vi "Create Sections and Channels.vi"(8 "error in (no error)":errorcluster, 10 "Configuration":T1={"Name"="", "Description"="", "Diagnostics Basic Configuraiton"={"Database File"=path "", "CAN Interface"=enum."CAN0", "Baud Rate"=0, "Diagnostic Protocol"=enum."GMLAN", "Transport Protocol"=enum."ISO TP - Normal Mode", "Transmit ID"=0, "Receive ID"=0, "Transmit Extension"=0, "Receive Extension"=0, "Receive UUDT ID"=0, "Enable Stream"=TRUE, "VW TP Channel ID"=0, "Security"={"Source DLL Path"=path "", "Security Level"=1, "Target DLL Path"=path ""}, "Fill Frame"=FALSE, "Fill Byte"=255, "Termination"=FALSE}, "DIDs"={"Description"="", "Frames"=[]}, "Input PIDs"={"Description"="", "Frames"=[]}, "Output PIDs"={"Description"="", "Frames"=[]}, "DPIDs"={"Description"="", "DPIDs"=[]}, "DTC"={"Description"="", "DTC descriptor"={"DTC Byte Length"=2, "Status Byte Length"=1, "Add Data Byte Length"=1, "Byte Order"=enum."Motorola"}, "DTCControl"={"Description"="", "Signals"=[]}}, "NI 986x Support"={"Enable 986x"=FALSE, "RIO Device"=0, "Bitfile"=path ""}, "Commands"={"Description"=""}, "Status"={"Description"=""}, "IO Controls"={"Description"="", "IO Control Array"=[]}, "Routines"={"Description"="", "Routine Array"=[]}, "Output Memory"={"Description"="", "Frames"=[]}, "Input Memory"={"Description"="", "Frames"=[]}} {"Input Memory"."Frames"."Signals"."Byte Order" items=["Little Endian", "Big Endian"]; "Input Memory"."Frames"."Signals"."Data Type" items=["Signed", "Unsigned", "IEEE Float"]; "Output Memory"."Frames"."Signals"."Byte Order" items=["Little Endian", "Big Endian"]; "Output Memory"."Frames"."Signals"."Data Type" items=["Signed", "Unsigned", "IEEE Float"]; "Routines"."Routine Array"."Stop Parameters"."Response"."Byte Order" items=["Little Endian", "Big Endian"]; "Routines"."Routine Array"."Stop Parameters"."Response"."Data Type" items=["Signed", "Unsigned", "IEEE Float"]; "Routines"."Routine Array"."Stop Parameters"."Cmd"."Byte Order" items=["Little Endian", "Big Endian"]; "Routines"."Routine Array"."Stop Parameters"."Cmd"."Data Type" items=["Signed", "Unsigned", "IEEE Float"]; "Routines"."Routine Array"."Request Parameters"."Response"."Byte Order" items=["Little Endian", "Big Endian"]; "Routines"."Routine Array"."Request Parameters"."Response"."Data Type" items=["Signed", "Unsigned", "IEEE Float"]; "Routines"."Routine Array"."Request Parameters"."Cmd"."Byte Order" items=["Little Endian", "Big Endian"]; "Routines"."Routine Array"."Request Parameters"."Cmd"."Data Type" items=["Signed", "Unsigned", "IEEE Float"]; "Routines"."Routine Array"."Start Parameters"."Response"."Byte Order" items=["Little Endian", "Big Endian"]; "Routines"."Routine Array"."Start Parameters"."Response"."Data Type" items=["Signed", "Unsigned", "IEEE Float"]; "Routines"."Routine Array"."Start Parameters"."Cmd"."Byte Order" items=["Little Endian", "Big Endian"]; "Routines"."Routine Array"."Start Parameters"."Cmd"."Data Type" items=["Signed", "Unsigned", "IEEE Float"]; "IO Controls"."IO Control Array"."Signals"."Response"."Byte Order" items=["Little Endian", "Big Endian"]; "IO Controls"."IO Control Array"."Signals"."Response"."Data Type" items=["Signed", "Unsigned", "IEEE Float"]; "IO Controls"."IO Control Array"."Signals"."Cmd"."Byte Order" items=["Little Endian", "Big Endian"]; "IO Controls"."IO Control Array"."Signals"."Cmd"."Data Type" items=["Signed", "Unsigned", "IEEE Float"]; "DTC"."DTCControl"."Signals"."Byte Order" items=["Little Endian", "Big Endian"]; "DTC"."DTCControl"."Signals"."Data Type" items=["Signed", "Unsigned", "IEEE Float"]; "Diagnostics Basic Configuraiton"."Fill Byte" format="%.0x"; "Diagnostics Basic Configuraiton"."VW TP Channel ID" format="%.0x"; "Diagnostics Basic Configuraiton"."Receive UUDT ID" format="%.0x"; "Diagnostics Basic Configuraiton"."Receive Extension" format="%.0x"; "Diagnostics Basic Configuraiton"."Transmit Extension" format="%.0x"; "Diagnostics Basic Configuraiton"."Receive ID" format="%.0x"; "Diagnostics Basic Configuraiton"."Transmit ID" format="%.0x"; "DIDs"."Frames"."Signals"."Byte Order" items=["Little Endian", "Big Endian"]; "DIDs"."Frames"."Signals"."Data Type" items=["Signed", "Unsigned", "IEEE Float"]; "Input PIDs"."Frames"."Signals"."Byte Order" items=["Little Endian", "Big Endian"]; "Input PIDs"."Frames"."Signals"."Data Type" items=["Signed", "Unsigned", "IEEE Float"]; "Output PIDs"."Frames"."Signals"."Byte Order" items=["Little Endian", "Big Endian"]; "Output PIDs"."Frames"."Signals"."Data Type" items=["Signed", "Unsigned", "IEEE Float"]}, 11 "Device Item Ref in":T25 format="%.0x") -> (0 "error out":errorcluster, 3 "Device Item Ref out":T25 format="%.0x")   [LabVIEW 2015, in "Diagnostics Addon System Explorer.lvlib"]
uses:
  Diagnostics Addon System Explorer.lvlib
  Types/FG Action.ctl
  <vilib>/NI Veristand/Custom Device API/Custom Device Channel.ctl
  <vilib>/NI Veristand/Custom Device API/Custom Device API.lvlib
  <vilib>/NI Veristand/Custom Device API/Custom Device Channel Type.ctl
  Shared/SubVIs/GUID Lookup.vi
  Shared/Diagnostics Addon Shared.lvlib
  Types/Frame Type.ctl
  Shared/Types/Signal Parameters.ctl
  <vilib>/NI Veristand/Custom Device API/Custom Device Item Ref.ctl
  Shared/Types/Diagnostic Protocols.ctl
  Shared/Types/CAN Interface.ctl
  Shared/Types/DPID Periodic Rate.ctl
  Shared/Types/DPID Parameters.ctl
  Types/Exported DPIDs Cluster.ctl
  Types/Exported Frames Cluster.ctl
  Shared/Types/Transport Protocols.ctl
  Shared/Types/CAN Configuration.ctl
  <vilib>/Automotive Diagnostic Command Set/Diagnostic Protocols.llb/DTC Descriptor.ctl
  Types/Exported DTC Cluster.ctl
  Types/Exported 986x Support.ctl
  Types/Exported Command Cluster.ctl
  Types/Exported Status Cluster.ctl
  Types/Exported Configuration.ctl
  Shared/Types/Frame Parameters.ctl
  Types/Exported DPID Parameters.ctl
  Shared/Types/Security.ctl
  Shared/Types/IO Control Parameters.ctl
  Shared/Types/Exported IO Control Cluster.ctl
  Shared/Types/Command Response Signals.ctl
  Shared/Types/Routine Paramaters.ctl
  Shared/Types/Exported Routines Cluster.ctl
  Shared/Types/Exported DTC Control Cluster.ctl
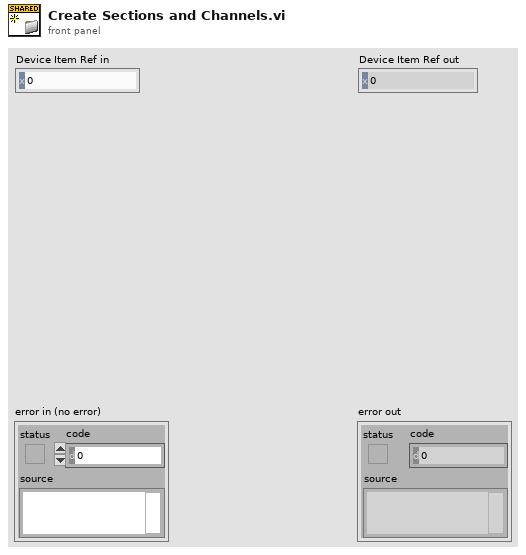
[diagram p1: front panel]
types:
  T1 = typedef "Diagnostics Addon System Explorer.lvlib/Exported Configuration.ctl" = cluster{"Name":string, "Description":string, "Diagnostics Basic Configuraiton":T2, "DIDs":T7, "Input PIDs":T7, "Output PIDs":T7, "DPIDs":T10, "DTC":T14, "NI 986x Support":T17, "Commands":T18, "Status":T19, "IO Controls":T20, "Routines":T23, "Output Memory":T7, "Input Memory":T7}
  T2 = typedef "Diagnostics Addon Shared.lvlib/CAN Configuration.ctl" = cluster{"Database File":path, "CAN Interface":T3, "Baud Rate":u32, "Diagnostic Protocol":T4, "Transport Protocol":T5, "Transmit ID":u32, "Receive ID":u32, "Transmit Extension":u8, "Receive Extension":u8, "Receive UUDT ID":u32, "Enable Stream":bool, "VW TP Channel ID":u32, "Security":T6, "Fill Frame":bool, "Fill Byte":u8, "Termination":bool}
  T3 = typedef "Diagnostics Addon Shared.lvlib/CAN Interface.ctl" = enum16{"CAN0", "CAN1", "CAN2", "CAN3", "CAN4", "CAN5", "CAN6", "CAN7", "CAN8", "CAN9", "CAN10", "CAN11", "CAN12", "CAN13", "CAN14", "CAN15", "CAN16", "CAN17", "CAN18", "CAN19", "CAN20", "CAN21", "CAN22", "CAN23", "CAN24", "CAN25", "CAN26", "CAN27", "CAN28", "CAN29", "CAN30", "CAN31", "CAN32", "CAN33", "CAN34", "CAN35", "CAN36", "CAN37", "CAN38", "CAN39", "CAN40", "CAN41", "CAN42", "CAN43", "CAN44", "CAN45", "CAN46", "CAN47", "CAN48", "CAN49", "CAN50", "CAN51", "CAN52", "CAN53", "CAN54", "CAN55", "CAN56", "CAN57", "CAN58", "CAN59", "CAN60", "CAN61", "CAN62", "CAN63", "CAN 256 (Virtual)", "CAN 257 (Virtual)"}
  T4 = typedef "Diagnostics Addon Shared.lvlib/Diagnostic Protocols.ctl" = enum16{"GMLAN", "KWP-2000", "UDS"}
  T5 = typedef "Diagnostics Addon Shared.lvlib/Transport Protocols.ctl" = enum16{"ISO TP - Normal Mode", "ISO TP - Mixed Mode", "VW TP 2.0", "Diagnostics on IP"}
  T6 = typedef "Diagnostics Addon Shared.lvlib/Security.ctl" = cluster{"Source DLL Path":path, "Security Level":u8, "Target DLL Path":path}
  T7 = typedef "Diagnostics Addon System Explorer.lvlib/Exported Frames Cluster.ctl" = cluster{"Description":string, "Frames":T8[]}
  T8 = typedef "Diagnostics Addon Shared.lvlib/Frame Parameters.ctl" = cluster{"Name":string, "Description":string, "ID":u32, "Signals":T9[]}
  T9 = typedef "Diagnostics Addon Shared.lvlib/Signal Parameters.ctl" = cluster{"Start Bit":u8, "Length":u8, "Scaling Factor":dbl, "Scaling Offset":dbl, "Minimum":dbl, "Maximum":dbl, "Data Type":u32, "Byte Order":u32, "Default Value":dbl, "Name":string, "Units":string, "Description":string}
  T10 = typedef "Diagnostics Addon System Explorer.lvlib/Exported DPIDs Cluster.ctl" = cluster{"Description":string, "DPIDs":T11[]}
  T11 = typedef "Diagnostics Addon System Explorer.lvlib/Exported DPID Parameters.ctl" = cluster{"Name":string, "Description":string, "DPID":T12}
  T12 = typedef "Diagnostics Addon Shared.lvlib/DPID Parameters.ctl" = cluster{"DPID ID":u8, "Speed":T13, "PIDs":u16[]}
  T13 = typedef "Diagnostics Addon Shared.lvlib/DPID Periodic Rate.ctl" = enum16{"Slow", "Medium", "Fast"}
  T14 = typedef "Diagnostics Addon System Explorer.lvlib/Exported DTC Cluster.ctl" = cluster{"Description":string, "DTC descriptor":T15, "DTCControl":T16}
  T15 = typedef "Diagnostics Addon Shared.lvlib/DTC Descriptor.ctl" = cluster{"DTC Byte Length":i32, "Status Byte Length":i32, "Add Data Byte Length":i32, "Byte Order":enum16{"Motorola", "Intel"}}
  T16 = typedef "Diagnostics Addon Shared.lvlib/Exported DTC Control Cluster.ctl" = cluster{"Description":string, "Signals":T9[]}
  T17 = typedef "Diagnostics Addon System Explorer.lvlib/Exported 986x Support.ctl" = cluster{"Enable 986x":bool, "RIO Device":u16, "Bitfile":path}
  T18 = typedef "Diagnostics Addon System Explorer.lvlib/Exported Command Cluster.ctl" = cluster{"Description":string}
  T19 = typedef "Diagnostics Addon System Explorer.lvlib/Exported Status Cluster.ctl" = cluster{"Description":string}
  T20 = typedef "Diagnostics Addon Shared.lvlib/Exported IO Control Cluster.ctl" = cluster{"Description":string, "IO Control Array":T21[]}
  T21 = typedef "Diagnostics Addon Shared.lvlib/IO Control Parameters.ctl" = cluster{"Name":string, "Description":string, "ID":u16, "Signals":T22}
  T22 = typedef "Diagnostics Addon Shared.lvlib/Command Response Signals.ctl" = cluster{"Cmd":T9[], "Response":T9[]}
  T23 = typedef "Diagnostics Addon Shared.lvlib/Exported Routines Cluster.ctl" = cluster{"Description":string, "Routine Array":T24[]}
  T24 = typedef "Diagnostics Addon Shared.lvlib/Routine Paramaters.ctl" = cluster{"Name":string, "Description":string, "ID":u16, "Start Parameters":T22, "Request Parameters":T22, "Stop Parameters":T22}
  T25 = typedef "Custom Device API.lvlib/Custom Device Item Ref.ctl" = u64
  T26 = typedef "Custom Device API.lvlib/Custom Device Channel.ctl" = cluster{"Type":T27, "Units":string, "Default Value":dbl, "Faultable":bool, "Scalable":bool}
  T27 = typedef "Custom Device API.lvlib/Custom Device Channel Type.ctl" = enum16{"Input", "Output"}
  T28 = typedef "Diagnostics Addon System Explorer.lvlib/FG Action.ctl" = enum16{"Get", "Set"}
  T29 = typedef "Diagnostics Addon System Explorer.lvlib/Frame Type.ctl" = enum8{"PID", "DID", "Memory"}
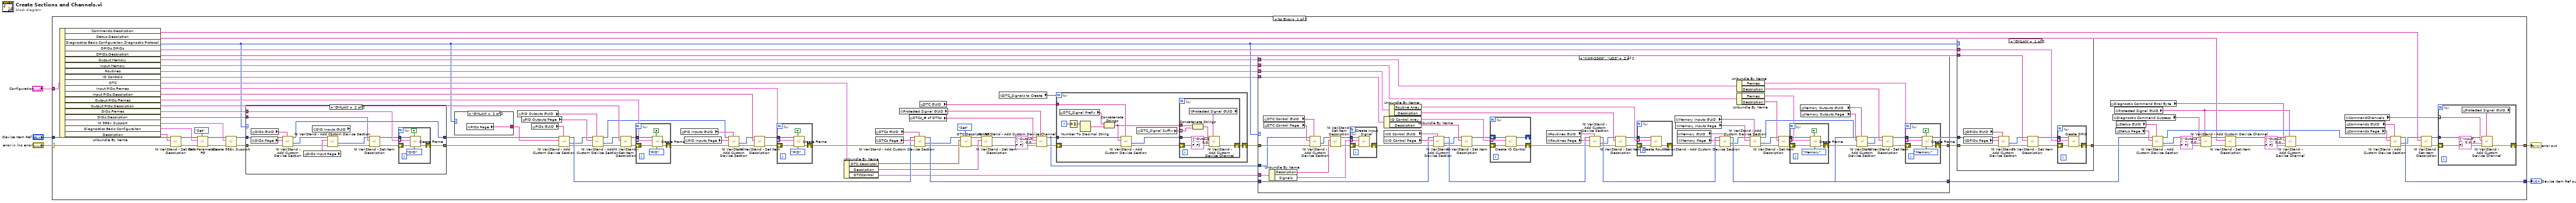
[diagram p0: block diagram]
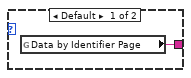
[diagram p3: hidden frame]
diagram:
  n1 = case shown="No Error" "error in (no error)" {
    selector: "error in (no error)" -> [w75 w274]
    tunnel: [w84 w274] -> w4
    tunnel: "Device Item Ref in" -> [w79 w273]
    tunnel: [w82 w273] -> w2
    tunnel: "Configuration" -> [w78 _]
    frame No Error {
      n2 = Unbundle By Name(w78) -> ("Commands.Description"=w52:string, "Status.Description"=w53:string, "Diagnostics Basic Configuraiton.Diagnostic Protocol"=w28:T4, "DPIDs.DPIDs"=w61:T11[], "DPIDs.Description"=w60:string, "Output Memory"=w21:T7, "Input Memory"=w20:T7, "Routines"=w22:T23, "IO Controls"=w23:T20, "DTC"=w65:T14, "Input PIDs.Frames"=w67:T8[], "Input PIDs.Description"=w68:string, "Output PIDs.Frames"=w66:T8[], "Output PIDs.Description"=w69:string, "DIDs.Frames"=w70:T8[], "DIDs.Description"=w71:string, "NI 986x Support"=w47:T17, "Diagnostics Basic Configuraiton"=w73:T2, "Description"=w74:string)
      n3 = call <vilib>:"NI VeriStand - Set Item Description.vi"("error in (no error)"=w75, "Description"=w74, "Item Ref in"=w79) -> ("error out"=w76:errorcluster, "Item Ref out"=w77:T25)  [unwired: 6 in, 1 out]
      n4 = call "CAN Parameters FG.vi"("Action"=FG_Action."Set", "error in (no error)"=w76, "Diagnostics Basic Configuraiton"=w73, "Device Item Ref in"=w77) -> ("error out"=w51:errorcluster, "Device Item Ref out"=w48:T25)  [unwired: 5 in, 1 out]
      n5 = call "Create 986x Support.vi"("error in (no error)"=w51, "986x Support"=w47, "Device Item Ref in"=w48) -> ("error out"=w50:errorcluster, "Device Ref out"=w49:T25)  [unwired: 7 in]
      n6 = case shown="\"GMLAN\"" w28 {
        tunnel: [w196 w210] -> w88
        tunnel: [w195 w209] -> w87
        tunnel: w71 -> [_ w197]
        tunnel: w70 -> [_ w208]
        tunnel: w50 -> [w196 w207]
        tunnel: w49 -> [w195 w206]
        frame Default {
        }
        frame "GMLAN" {
          n7 = global read "GUID Lookup.vi" "DIDs GUID"() -> (w211:string)
          n8 = global read "GUID Lookup.vi" "DIDs Page"() -> (w212:string)
          n9 = call <vilib>:"NI VeriStand - Add Custom Device Section.vi"("GUID (Default Section)"=w211, "error in (no error)"=w207, "Section Name"=w212, "Parent Ref in"=w206) -> ("error out"=w199:errorcluster, "Section Ptr"=w198:T25, "Parent Ref out"=w209:T25)  [unwired: 4 in, 1 out]
          n10 = global read "GUID Lookup.vi" "DIDs Input Page"() -> (w204:string)
          n11 = global read "GUID Lookup.vi" "DID Inputs GUID"() -> (w205:string)
          n12 = call <vilib>:"NI VeriStand - Add Custom Device Section.vi"("GUID (Default Section)"=w205, "error in (no error)"=w199, "Section Name"=w204, "Parent Ref in"=w198) -> ("error out"=w203:errorcluster, "Section Ptr"=w202:T25)  [unwired: 4 in, 2 out]
          n13 = call <vilib>:"NI VeriStand - Set Item Description.vi"("error in (no error)"=w203, "Description"=w197, "Item Ref in"=w202) -> ("error out"=w201:errorcluster, "Item Ref out"=w200:T25)  [unwired: 6 in, 1 out]
          n14 = for {
            tunnel: w200 -> [w214]
            shift-right: [w213] -> w210
            shift-left: w201 -> [w216]
            tunnel: w208 -> [w215] mode=indexing
            n15 = call "Create Frame.vi"("Type"=Frame_Type."DID", "Input?"=TRUE, "error in (no error)"=w216, "Frame"=w215, "Section Ptr"=w214) -> ("error out"=w213:errorcluster)  [unwired: 5 in, 1 out]
          }
        }
      }
      n16 = case shown="\"GMLAN\"" w28 {
        tunnel: [w193 w194] -> w45
        frame Default {
          n17 = global read "GUID Lookup.vi" "Data by Identifier Page"() -> (w193:string)
        }
        frame "GMLAN" {
          n18 = global read "GUID Lookup.vi" "PIDs Page"() -> (w194:string)
        }
      }
      n19 = global read "GUID Lookup.vi" "PID Outputs GUID"() -> (w42:string)
      n20 = global read "GUID Lookup.vi" "PID Outputs Page"() -> (w41:string)
      n21 = global read "GUID Lookup.vi" "PIDs GUID"() -> (w46:string)
      n22 = call <vilib>:"NI VeriStand - Add Custom Device Section.vi"("GUID (Default Section)"=w46, "error in (no error)"=w88, "Section Name"=w45, "Parent Ref in"=w87) -> ("error out"=w40:errorcluster, "Section Ptr"=w39:T25, "Parent Ref out"=w101:T25)  [unwired: 4 in, 1 out]
      n23 = call <vilib>:"NI VeriStand - Add Custom Device Section.vi"("GUID (Default Section)"=w42, "error in (no error)"=w40, "Section Name"=w41, "Parent Ref in"=w39) -> ("error out"=w38:errorcluster, "Section Ptr"=w33:T25, "Parent Ref out"=w29:T25)  [unwired: 4 in, 1 out]
      n24 = call <vilib>:"NI VeriStand - Set Item Description.vi"("error in (no error)"=w38, "Description"=w69, "Item Ref in"=w33) -> ("error out"=w31:errorcluster, "Item Ref out"=w32:T25)  [unwired: 6 in, 1 out]
      n25 = for {
        tunnel: w32 -> [w222]
        shift-right: [w223] -> w30
        shift-left: w31 -> [w224]
        tunnel: w66 -> [w221] mode=indexing
        n26 = call "Create Frame.vi"("Type"=Frame_Type."PID", "Input?"=FALSE, "error in (no error)"=w224, "Frame"=w221, "Section Ptr"=w222) -> ("error out"=w223:errorcluster)  [unwired: 5 in, 1 out]
      }
      n27 = global read "GUID Lookup.vi" "PID Inputs GUID"() -> (w44:string)
      n28 = global read "GUID Lookup.vi" "PID Inputs Page"() -> (w43:string)
      n29 = call <vilib>:"NI VeriStand - Add Custom Device Section.vi"("GUID (Default Section)"=w44, "error in (no error)"=w30, "Section Name"=w43, "Parent Ref in"=w29) -> ("error out"=w37:errorcluster, "Section Ptr"=w35:T25)  [unwired: 4 in, 2 out]
      n30 = call <vilib>:"NI VeriStand - Set Item Description.vi"("error in (no error)"=w37, "Description"=w68, "Item Ref in"=w35) -> ("error out"=w36:errorcluster, "Item Ref out"=w34:T25)  [unwired: 6 in, 1 out]
      n31 = for {
        tunnel: w34 -> [w228]
        shift-right: [w229] -> w102
        shift-left: w36 -> [w230]
        tunnel: w67 -> [w227] mode=indexing
        n32 = call "Create Frame.vi"("Type"=Frame_Type."PID", "Input?"=TRUE, "error in (no error)"=w230, "Frame"=w227, "Section Ptr"=w228) -> ("error out"=w229:errorcluster)  [unwired: 5 in, 1 out]
      }
      n33 = Unbundle By Name(w65) -> ("DTC descriptor"=w14:T15, "Description"=w62:string, "DTCControl"=w12:T16)
      n34 = global read "GUID Lookup.vi" "DTCs GUID"() -> (w103:string)
      n35 = global read "GUID Lookup.vi" "DTCs Page"() -> (w104:string)
      n36 = global read "GUID Lookup.vi" "Protected Signal GUID"() -> (w80:string)
      n37 = global read "GUID Lookup.vi" "DTCs_# of DTCs"() -> (w99:string)
      n38 = call <vilib>:"NI VeriStand - Add Custom Device Section.vi"("GUID (Default Section)"=w103, "error in (no error)"=w102, "Section Name"=w104, "Parent Ref in"=w101) -> ("error out"=w18:errorcluster, "Section Ptr"=w19:T25, "Parent Ref out"=w26:T25)  [unwired: 4 in, 1 out]
      n39 = global read "GUID Lookup.vi" "DTC GUID"() -> (w90:string)
      n40 = call "DTC Descriptor FG.vi"("Action"=FG_Action."Set", "error in (no error)"=w18, "DTC descriptor"=w14, "Device Item Ref in"=w19) -> ("error out"=w17:errorcluster, "Device Item Ref out"=w16:T25)  [unwired: 5 in, 1 out]
      n41 = call <vilib>:"NI VeriStand - Set Item Description.vi"("error in (no error)"=w17, "Description"=w62, "Item Ref in"=w16) -> ("error out"=w64:errorcluster, "Item Ref out"=w63:T25)  [unwired: 6 in, 1 out]
      n42 = global read "GUID Lookup.vi" "DTC_Signals to Create"() -> (w89:i32)
      n43 = call <vilib>:"NI VeriStand - Add Custom Device Channel.vi"("GUID (Default Channel)"=w80, "error in (no error)"=w64, "Channel"=T26 {"Type"=enum."Output", "Units"="", "Default Value"=0.0, "Faultable"=FALSE, "Scalable"=FALSE}, "Channel Name"=w99, "Parent Ref in"=w63) -> ("error out"=w91:errorcluster, "Parent Ref out"=w13:T25)  [unwired: 3 in, 2 out]
      n44 = for {
        N: w89 -> [_]
        tunnel: w13 -> [w260]
        shift-right: [w264] -> w27
        shift-left: w91 -> [w258]
        tunnel: w90 -> [w255]
        i -> [w263]
        n45 = global read "GUID Lookup.vi" "DTC_Signal Prefix"() -> (w253:string)
        n46 = Increment(x=w263) -> (x+1=w262:i32)
        n47 = Number To Decimal String(number=w262) -> (decimal integer string=w261:string)  [unwired: 1 in]
        n48 = Concatenate Strings(w253, w261) -> (w256:string)
        n49 = call <vilib>:"NI VeriStand - Add Custom Device Section.vi"("GUID (Default Section)"=w255, "error in (no error)"=w258, "Section Name"=w256, "Parent Ref in"=w260) -> ("error out"=w257:errorcluster, "Section Ptr"=w259:T25)  [unwired: 4 in, 2 out]
        n50 = global read "GUID Lookup.vi" "DTC_Signal Suffix"() -> (w254:string[])
        n51 = for {
          tunnel: w259 -> [w270]
          tunnel: w256 -> [w267]
          tunnel: w254 -> [w268] mode=indexing
          shift-right: [w272] -> w264
          shift-left: w257 -> [w269]
          n52 = global read "GUID Lookup.vi" "Protected Signal GUID"() -> (w265:string)
          n53 = Concatenate Strings(w267, w268) -> (w266:string)
          n54 = call <vilib>:"NI VeriStand - Add Custom Device Channel.vi"("GUID (Default Channel)"=w265, "error in (no error)"=w269, "Channel"=T26 {"Type"=enum."Output", "Units"="", "Default Value"=0.0, "Faultable"=FALSE, "Scalable"=FALSE}, "Channel Name"=w266, "Parent Ref in"=w270) -> ("error out"=w272:errorcluster)  [unwired: 3 in, 3 out]
        }
      }
      n55 = case shown="\"KWP-2000\", \"UDS\"" w28 {
        tunnel: w27 -> [w105 w118]
        tunnel: w26 -> [w106 w154]
        tunnel: [w106 w142] -> w25
        tunnel: [w105 w127] -> w24
        tunnel: w23 -> [_ w162]
        tunnel: w22 -> [_ w149]
        tunnel: w21 -> [_ w121]
        tunnel: w20 -> [_ w124]
        tunnel: w13 -> [_ w117]
        tunnel: w12 -> [_ w111]
        frame "GMLAN" {
        }
        frame "KWP-2000", "UDS" {
          n56 = global read "GUID Lookup.vi" "DTC Control GUID"() -> (w107:string)
          n57 = global read "GUID Lookup.vi" "DTC Control Page"() -> (w108:string)
          n58 = Unbundle By Name(w111) -> ("Description"=w110:string, "Signals"=w109:T9[])
          n59 = call <vilib>:"NI VeriStand - Add Custom Device Section.vi"("GUID (Default Section)"=w107, "error in (no error)"=w118, "Section Name"=w108, "Parent Ref in"=w117) -> ("error out"=w113:errorcluster, "Section Ptr"=w115:T25)  [unwired: 4 in, 2 out]
          n60 = call <vilib>:"NI VeriStand - Set Item Description.vi"("error in (no error)"=w113, "Description"=w110, "Item Ref in"=w115) -> ("error out"=w112:errorcluster, "Item Ref out"=w114:T25)  [unwired: 6 in, 1 out]
          n61 = for {
            shift-right: [w170] -> w116
            shift-left: w112 -> [w171]
            tunnel: w109 -> [w168] mode=indexing
            tunnel: w114 -> [w169]
            n62 = call "Create Input Signal.vi"("error in (no error)"=w171, "Signal Parameters"=w168, "Section Ptr"=w169) -> ("error out"=w170:errorcluster)  [unwired: 7 in, 1 out]
          }
          n63 = global read "GUID Lookup.vi" "IO Control GUID"() -> (w160:string)
          n64 = Unbundle By Name(w162) -> ("IO Control Array"=w161:T21[], "Description"=w152:string)
          n65 = global read "GUID Lookup.vi" "IO Control Page"() -> (w159:string)
          n66 = Unbundle By Name(w149) -> ("Routine Array"=w148:T24[], "Description"=w147:string)
          n67 = call <vilib>:"NI VeriStand - Add Custom Device Section.vi"("GUID (Default Section)"=w160, "error in (no error)"=w116, "Section Name"=w159, "Parent Ref in"=w154) -> ("error out"=w158:errorcluster, "Section Ptr"=w157:T25, "Parent Ref out"=w153:T25)  [unwired: 4 in, 1 out]
          n68 = call <vilib>:"NI VeriStand - Set Item Description.vi"("error in (no error)"=w158, "Description"=w152, "Item Ref in"=w157) -> ("error out"=w156:errorcluster, "Item Ref out"=w155:T25)  [unwired: 6 in, 1 out]
          n69 = for {
            shift-right: [w191] -> w163
            shift-left: w156 -> [w192]
            shift-right: [w189] -> _
            shift-left: w155 -> [w190]
            tunnel: w161 -> [w188] mode=indexing
            n70 = call "Create IO Control.vi"("error in (no error)"=w192, "IO Control"=w188, "Section Ptr"=w190) -> ("error out"=w191:errorcluster, "Parent Ref out"=w189:T25)  [unwired: 7 in]
          }
          n71 = global read "GUID Lookup.vi" "Routines GUID"() -> (w164:string)
          n72 = global read "GUID Lookup.vi" "Routines Page"() -> (w165:string)
          n73 = call <vilib>:"NI VeriStand - Add Custom Device Section.vi"("GUID (Default Section)"=w164, "error in (no error)"=w163, "Section Name"=w165, "Parent Ref in"=w153) -> ("error out"=w166:errorcluster, "Section Ptr"=w167:T25, "Parent Ref out"=w143:T25)  [unwired: 4 in, 1 out]
          n74 = call <vilib>:"NI VeriStand - Set Item Description.vi"("error in (no error)"=w166, "Description"=w147, "Item Ref in"=w167) -> ("error out"=w151:errorcluster, "Item Ref out"=w150:T25)  [unwired: 6 in, 1 out]
          n75 = for {
            shift-right: [w186] -> w144
            shift-left: w151 -> [w187]
            tunnel: w150 -> [w185]
            tunnel: w148 -> [w184] mode=indexing
            n76 = call "Create Routine.vi"("error in (no error)"=w187, "Routine"=w184, "Section Ptr"=w185) -> ("error out"=w186:errorcluster)  [unwired: 7 in, 1 out]
          }
          n77 = global read "GUID Lookup.vi" "Memory Inputs GUID"() -> (w141:string)
          n78 = global read "GUID Lookup.vi" "Memory Inputs Page"() -> (w140:string)
          n79 = global read "GUID Lookup.vi" "Memory GUID"() -> (w146:string)
          n80 = global read "GUID Lookup.vi" "Memory Page"() -> (w145:string)
          n81 = call <vilib>:"NI VeriStand - Add Custom Device Section.vi"("GUID (Default Section)"=w146, "error in (no error)"=w144, "Section Name"=w145, "Parent Ref in"=w143) -> ("error out"=w126:errorcluster, "Section Ptr"=w125:T25, "Parent Ref out"=w142:T25)  [unwired: 4 in, 1 out]
          n82 = Unbundle By Name(w121) -> ("Frames"=w120:T8[], "Description"=w119:string)
          n83 = Unbundle By Name(w124) -> ("Frames"=w122:T8[], "Description"=w123:string)
          n84 = call <vilib>:"NI VeriStand - Add Custom Device Section.vi"("GUID (Default Section)"=w141, "error in (no error)"=w126, "Section Name"=w140, "Parent Ref in"=w125) -> ("error out"=w139:errorcluster, "Section Ptr"=w134:T25, "Parent Ref out"=w130:T25)  [unwired: 4 in, 1 out]
          n85 = call <vilib>:"NI VeriStand - Set Item Description.vi"("error in (no error)"=w139, "Description"=w123, "Item Ref in"=w134) -> ("error out"=w132:errorcluster, "Item Ref out"=w133:T25)  [unwired: 6 in, 1 out]
          n86 = for {
            tunnel: w133 -> [w175]
            shift-right: [w176] -> w131
            shift-left: w132 -> [w177]
            tunnel: w122 -> [w174] mode=indexing
            n87 = call "Create Frame.vi"("Type"=Frame_Type."Memory", "Input?"=TRUE, "error in (no error)"=w177, "Frame"=w174, "Section Ptr"=w175) -> ("error out"=w176:errorcluster)  [unwired: 5 in, 1 out]
          }
          n88 = global read "GUID Lookup.vi" "Memory Outputs GUID"() -> (w128:string)
          n89 = global read "GUID Lookup.vi" "Memory Outputs Page"() -> (w129:string)
          n90 = call <vilib>:"NI VeriStand - Add Custom Device Section.vi"("GUID (Default Section)"=w128, "error in (no error)"=w131, "Section Name"=w129, "Parent Ref in"=w130) -> ("error out"=w138:errorcluster, "Section Ptr"=w136:T25)  [unwired: 4 in, 2 out]
          n91 = call <vilib>:"NI VeriStand - Set Item Description.vi"("error in (no error)"=w138, "Description"=w119, "Item Ref in"=w136) -> ("error out"=w137:errorcluster, "Item Ref out"=w135:T25)  [unwired: 6 in, 1 out]
          n92 = for {
            tunnel: w135 -> [w181]
            shift-right: [w182] -> w127
            shift-left: w137 -> [w183]
            tunnel: w120 -> [w180] mode=indexing
            n93 = call "Create Frame.vi"("Type"=Frame_Type."Memory", "Input?"=FALSE, "error in (no error)"=w183, "Frame"=w180, "Section Ptr"=w181) -> ("error out"=w182:errorcluster)  [unwired: 5 in, 1 out]
          }
        }
      }
      n94 = case shown="\"GMLAN\"" w28 {
        tunnel: [w243 w252] -> w98
        tunnel: w24 -> [w245 w252]
        tunnel: w25 -> [w244 _]
        tunnel: w61 -> [w242 _]
        tunnel: w60 -> [w237 _]
        frame "GMLAN" {
          n95 = global read "GUID Lookup.vi" "DPIDs GUID"() -> (w247:string)
          n96 = global read "GUID Lookup.vi" "DPIDs Page"() -> (w246:string)
          n97 = call <vilib>:"NI VeriStand - Add Custom Device Section.vi"("GUID (Default Section)"=w247, "error in (no error)"=w245, "Section Name"=w246, "Parent Ref in"=w244) -> ("error out"=w241:errorcluster, "Section Ptr"=w239:T25)  [unwired: 4 in, 2 out]
          n98 = call <vilib>:"NI VeriStand - Set Item Description.vi"("error in (no error)"=w241, "Description"=w237, "Item Ref in"=w239) -> ("error out"=w240:errorcluster, "Item Ref out"=w238:T25)  [unwired: 6 in, 1 out]
          n99 = for {
            tunnel: w238 -> [w249]
            shift-right: [w250] -> w243
            shift-left: w240 -> [w251]
            tunnel: w242 -> [w248] mode=indexing
            n100 = call "Create DPID.vi"("error in (no error)"=w251, "DPID"=w248, "Section Ptr"=w249) -> ("error out"=w250:errorcluster)  [unwired: 7 in, 1 out]
          }
        }
        frame Default {
        }
      }
      n101 = global read "GUID Lookup.vi" "Diagnostic Command Error Byte"() -> (w6:string)
      n102 = global read "GUID Lookup.vi" "Diagnostic Command Success"() -> (w92:string)
      n103 = global read "GUID Lookup.vi" "Protected Signal GUID"() -> (w7:string)
      n104 = global read "GUID Lookup.vi" "Status Page"() -> (w96:string)
      n105 = global read "GUID Lookup.vi" "Status GUID"() -> (w97:string)
      n106 = call <vilib>:"NI VeriStand - Add Custom Device Section.vi"("GUID (Default Section)"=w97, "error in (no error)"=w98, "Section Name"=w96, "Parent Ref in"=w25) -> ("error out"=w93:errorcluster, "Section Ptr"=w94:T25, "Parent Ref out"=w83:T25)  [unwired: 4 in, 1 out]
      n107 = call <vilib>:"NI VeriStand - Add Custom Device Channel.vi"("GUID (Default Channel)"=w7, "error in (no error)"=w93, "Channel"=T26 {"Type"=enum."Output", "Units"="", "Default Value"=0.0, "Faultable"=FALSE, "Scalable"=FALSE}, "Channel Name"=w92, "Parent Ref in"=w94) -> ("error out"=w58:errorcluster, "Parent Ref out"=w59:T25)  [unwired: 3 in, 2 out]
      n108 = call <vilib>:"NI VeriStand - Set Item Description.vi"("error in (no error)"=w58, "Description"=w53, "Item Ref in"=w59) -> ("error out"=w10:errorcluster, "Item Ref out"=w9:T25)  [unwired: 6 in, 1 out]
      n109 = call <vilib>:"NI VeriStand - Add Custom Device Channel.vi"("GUID (Default Channel)"=w7, "error in (no error)"=w10, "Channel"=T26 {"Type"=enum."Output", "Units"="", "Default Value"=0.0, "Faultable"=FALSE, "Scalable"=FALSE}, "Channel Name"=w6, "Parent Ref in"=w9) -> ("error out"=w8:errorcluster)  [unwired: 3 in, 3 out]
      n110 = global read "GUID Lookup.vi" "CommandChannels"() -> (w81:string[])
      n111 = global read "GUID Lookup.vi" "Commands GUID"() -> (w85:string)
      n112 = global read "GUID Lookup.vi" "Commands Page"() -> (w86:string)
      n113 = call <vilib>:"NI VeriStand - Add Custom Device Section.vi"("GUID (Default Section)"=w85, "error in (no error)"=w8, "Section Name"=w86, "Parent Ref in"=w83) -> ("error out"=w57:errorcluster, "Section Ptr"=w55:T25, "Parent Ref out"=w82:T25)  [unwired: 4 in, 1 out]
      n114 = call <vilib>:"NI VeriStand - Set Item Description.vi"("error in (no error)"=w57, "Description"=w52, "Item Ref in"=w55) -> ("error out"=w56:errorcluster, "Item Ref out"=w54:T25)  [unwired: 6 in, 1 out]
      n115 = for {
        tunnel: w81 -> [w236] mode=indexing
        tunnel: w54 -> [w234]
        shift-right: [w232] -> w84
        shift-left: w56 -> [w235]
        n116 = global read "GUID Lookup.vi" "Protected Signal GUID"() -> (w231:string)
        n117 = call <vilib>:"NI VeriStand - Add Custom Device Channel.vi"("GUID (Default Channel)"=w231, "error in (no error)"=w235, "Channel"=T26 {"Type"=enum."Input", "Units"="", "Default Value"=0.0, "Faultable"=FALSE, "Scalable"=FALSE}, "Channel Name"=w236, "Parent Ref in"=w234) -> ("error out"=w232:errorcluster)  [unwired: 3 in, 3 out]
      }
    }
    frame Error {
    }
  }
  "error out" <- w4
  "Device Item Ref out" <- w2
